vi "Launch.vi"(8 "error in":errorcluster, 11 "Flex UI in":refnum<class "Flex UI.lvclass">) -> (0 "error out":errorcluster, 3 "Flex UI out":refnum<class "Flex UI.lvclass">)   [LabVIEW 2016, in "Flex UI.lvclass"]
doc: "Launches the UI."
uses:
  Flex UI.lvclass
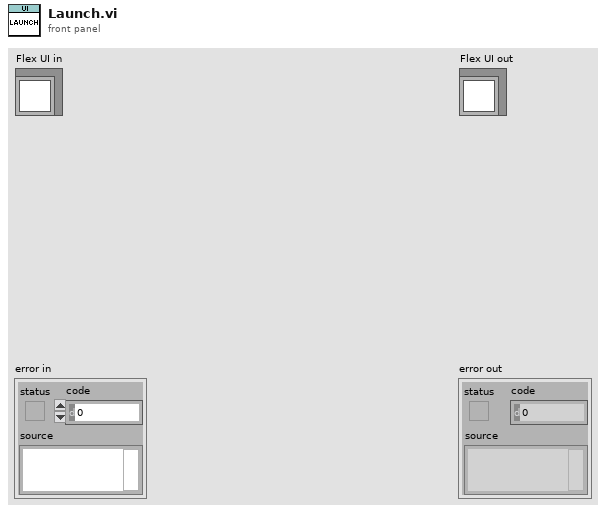
[diagram p1: front panel]
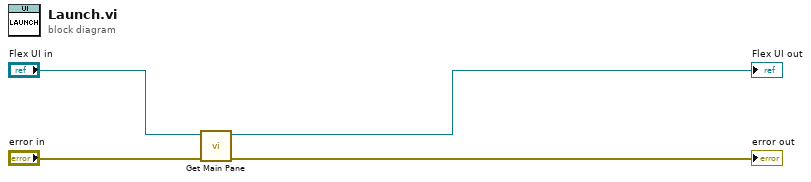
[diagram p0: block diagram]
diagram:
  n1 = call-dynamic "Get Main Pane.vi"("error in"="error in", "Flex UI in"="Flex UI in") -> ("error out"=→"error out":errorcluster, "Flex UI out"=→"Flex UI out":refnum<class "Flex UI.lvclass">)  [unwired: 8 in]
